vi "ConfigMultiPoint.vi"(8 "error in (no error)":errorcluster, 11 "NiPxi6123 in":refnum<class "NiPxi6123.lvclass">) -> (0 "error out":errorcluster, 3 "NiPxi6123 out":refnum<class "NiPxi6123.lvclass">)   [LabVIEW 2014, in "SamplerPlugins.lvlib" / "NiPxi6123.lvclass"]
uses:
  NiPxi6123.lvclass
  <vilib>/DAQmx/create/channels.llb/DAQmx Create Channel (AI-Voltage-Basic).vi
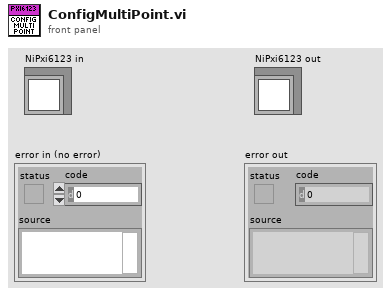
[diagram p1: front panel]
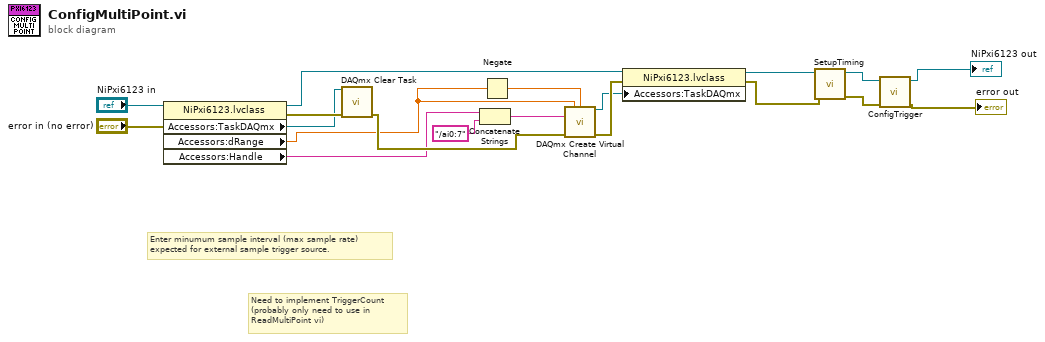
[diagram p0: block diagram]
diagram:
  # "Enter minumum sample interval (max sample rate) \nexpected for external sample trigger source."
  # "Need to implement TriggerCount\n(probably only need to use in\nReadMultiPoint vi)"
  n1 = property class="NiPxi6123.lvclass"(reference="NiPxi6123 in", error in="error in (no error)") -> (reference out=w12:refnum<class "NiPxi6123.lvclass">, error out=w14:errorcluster, "Accessors:TaskDAQmx"=w3:refnum<k21>, "Accessors:dRange"=w2:dbl, "Accessors:Handle"=w1:string)
  n2 = call <vilib>:"DAQmx Clear Task.vi"("task in"=w3, "error in"=w14) -> ("error out"=w13:errorcluster)  [unwired: 13 in]
  n3 = Concatenate Strings(w1, "/ai0:7" ("regular expression")) -> (w15:string)
  n4 = Negate(x=w2) -> (-x=w17:dbl)
  n5 = call-poly <vilib>:"DAQmx Create Virtual Channel.vi"("maximum value"=w2, "minimum value"=w17, "physical channels"=w15, "error in"=w13) -> ("task out"=w10:refnum<k21>, "error out"=w11:errorcluster)  [unwired: 10 in]
  n6 = property class="NiPxi6123.lvclass"(reference=w12, error in=w11, "Accessors:TaskDAQmx"=w10) -> (reference out=w7:refnum<class "NiPxi6123.lvclass">, error out=w6:errorcluster)
  n7 = call "SetupTiming.vi"("error in (no error)"=w6, "ClassIn"=w7) -> ("error out"=w8:errorcluster, "ClassOut"=w9:refnum<class "NiPxi6123.lvclass">)  [unwired: 8 in]
  n8 = call-dynamic "ConfigTrigger.vi"("error in (no error)"=w8, "NiPxi6123 in"=w9) -> ("error out"=→"error out":errorcluster, "NiPxi6123 out"=→"NiPxi6123 out":refnum<class "NiPxi6123.lvclass">)  [unwired: 8 in]
